vi "macro_LinearFilter_ExecuteTC.vi"   [LabVIEW 2019, in "Trajectory_Library.lvlib"]
uses:
  Trajectory_Library.lvlib
types:
  T1 = enum16{"Moving Average", "Low Pass 1st Order Butterworth", "Low Pass 2nd Order Butterworth", "High Pass 1st Order Butterworth", "High Pass 2nd Order Butterworth"}
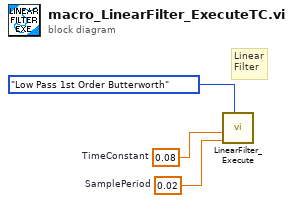
[diagram p0: block diagram]
diagram:
  w1 = 0.02  # SamplePeriod
  w2 = 0.08  # TimeConstant
  # "Linear\nFilter"
  n1 = call "LinearFilter_Execute.vi"("Filter Type"=T1."Low Pass 1st Order Butterworth", "SamplePeriod"=w1, "TimeConstant"=w2) -> ()  [unwired: 7 in, 2 out]
